vi "Get Pin Number.vi"(11 "pin number":T1 items=["D0"=0, "D1"=1, "D2"=2, "D3"=3, "D4"=4, "D5"=5, "D6"=6, "D7"=7, "D8"=8, "D9"=9, "D10"=10, "D11"=11, "D12"=12, "D13"=13, "D14"=14, "D15"=15, "LED_BUILTIN"=1001]) -> (3 "String":string)   [LabVIEW 2014]
uses:
  Basic API/ctl/digitalPin.ctl
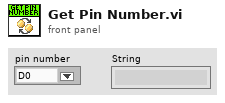
[diagram p1: front panel]
types:
  T1 = typedef "digitalPin.ctl" = u16
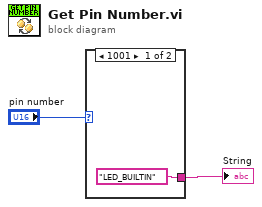
[diagram p0: block diagram]
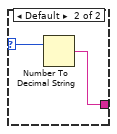
[diagram p2: hidden frame]
diagram:
  n1 = case shown="1001" "pin number" {
    selector: "pin number" -> [_ w4]
    tunnel: ["LED_BUILTIN" w5] -> w1
    frame 1001 {
    }
    frame Default {
      n2 = Number To Decimal String(number=w4) -> (decimal integer string=w5:string)  [unwired: 1 in]
    }
  }
  "String" <- w1
